vi "Target.vi"() -> ()   [LabVIEW 2018]
uses:
  <vilib>/rvi/Emulation/niFpgaGetClockAttributes.vi
  <vilib>/rvi/Emulation/niFpgaSctlEmulationGetInTimedLoop.vi
  <vilib>/rvi/Emulation/niFpgaEmulationReportErrorSimple.vi
  <vilib>/rvi/eio/common/nirviEmuTemplateMethod_errors.vi
  <vilib>/rvi/Emulation/niFpgaCriticalErrorInLSC.vi
  <vilib>/eio/EIONode/EIONode.xnode
panel:
  out "DAT":bool[](array[boolean])
  in  "CLK":i32=20
  in  "CLKDAT ticks":u16=40 caption="Count(Ticks)"
  in  "CLKDAT":bool
  in  "Частота":bool
  out "MISO":bool[](array[boolean])
  in  "Offset":i16=-1
  in  "phase offset N":fxp<+,32,0>=0.25
  in  "frequency N":fxp<+,32,0>=2.491287887096405e-08
  in  "phase offset P":fxp<+,32,0>
  in  "frequency P":fxp<+,32,0>=2.491287887096405e-08
  in  "N (24/16)":i32=24
  in  "MOSI":bool[](array[boolean])=[FALSE, FALSE, FALSE, FALSE, FALSE, FALSE, FALSE, FALSE, FALSE, FALSE, FALSE, FALSE, FALSE, FALSE, FALSE, FALSE, FALSE, FALSE, FALSE, FALSE, FALSE, FALSE, FALSE, FALSE]
  in  "Count(Ticks)":u16=40
  in  "NPRG":bool
  out "NERR":bool
  out "INCB":bool
  out "INCA":bool
  out "B":bool
  out "A":bool
  out "Z":bool
  out "INCZ":bool
  out "PSIN":i16
  out "POK":i16
  out "ERR":i16
  out "NCOS":i16
  out "NSIN":i16
  out "PCOS":i16
  in  "Регистр":bool
  in  "Стоп":bool
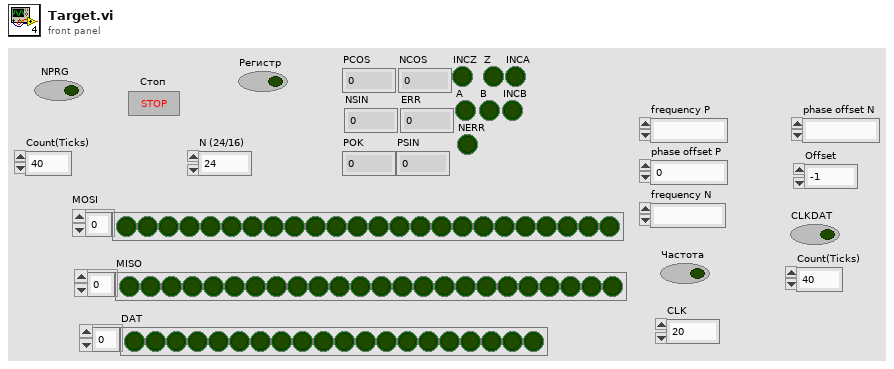
[diagram p1: front panel]
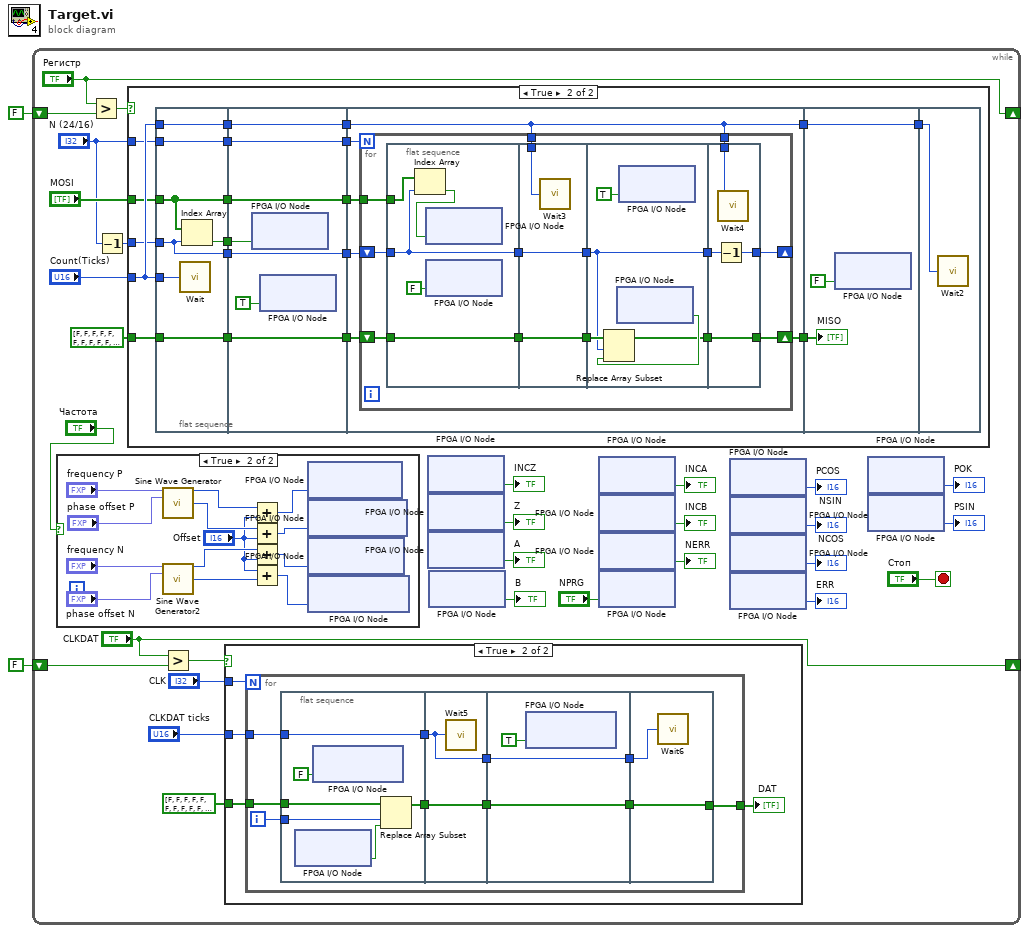
[diagram p0: block diagram]
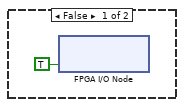
[diagram p2: hidden frame]
diagram:
  n1 = while {
    shift-right: ["CLKDAT"] -> _
    shift-left: FALSE ("CLKDAT") -> [w8]
    shift-right: ["Регистр"] -> _
    shift-left: FALSE ("Регистр") -> [w5]
    stop <- "Стоп" stop-if-true
    n2 = case shown="True" "Частота" {
      frame False {
      }
      frame True {
        n3 = call "Sine Wave Generator"("frequency (periods/tick)"="frequency P", "phase offset (periods)"="phase offset P") -> ("sine out"=w69:i16, "cosine out"=w68:i16)  [unwired: 12 in]
        n4 = call "Sine Wave Generator2"("frequency (periods/tick)"="frequency N", "phase offset (periods)"="phase offset N") -> ("sine out"=w67:i16, "cosine out"=w66:i16)  [unwired: 12 in]
        n5 = Add(x=w69, y="Offset") -> (x+y=w64:i16)
        n6 = Add(x=w68, y="Offset") -> (x+y=w63:i16)
        n7 = Add(x=w67, y="Offset") -> (x+y=w62:i16)
        n8 = Add(x="Offset", y=w66) -> (x+y=w61:i16)
        n9 = xnode "FPGA I/O Node"("PSIN_NQI"=w64) -> ()  [unwired: 1 in, 1 out]
        n10 = xnode "FPGA I/O Node"("PCOS_NQI"=w63) -> ()  [unwired: 1 in, 1 out]
        n11 = xnode "FPGA I/O Node"("NSIN_NQI"=w62) -> ()  [unwired: 1 in, 1 out]
        n12 = xnode "FPGA I/O Node"("NCOS_NQI"=w61) -> ()  [unwired: 1 in, 1 out]
      }
    }
    n13 = Greater?(x="Регистр", y=w5) -> (0:w3:bool)
    n14 = Decrement(x="N (24/16)") -> (x-1=w13:i32)
    n15 = case shown="True" w3 {
      tunnel: "Count(Ticks)" -> [_ w92]
      tunnel: w13 -> [_ w91]
      tunnel: "MOSI" -> [_ w90]
      tunnel: bool[] [FALSE, FALSE, FALSE, FALSE, FALSE, FALSE, FALSE, FALSE, FALSE, FALSE, FALSE, FALSE, FALSE, FALSE, FALSE, FALSE, FALSE, FALSE, FALSE, FALSE, FALSE, FALSE, FALSE, FALSE] ("MISO") -> [_ w89]
      tunnel: "N (24/16)" -> [_ w76]
      frame False {
      }
      frame True {
        n16 = flat-sequence {
          tunnel: w92 -> [w99]
          tunnel: [w98] -> w88
          tunnel: w92 -> [w98]
          tunnel: [w97] -> w87
          tunnel: w91 -> [w96]
          tunnel: [w96] -> w86
          tunnel: w90 -> [w95]
          tunnel: [w95] -> w85
          tunnel: [w94] -> w84
          tunnel: w89 -> [w94]
          tunnel: [w93] -> w77
          tunnel: w76 -> [w93]
          tunnel: [w105] -> w83
          tunnel: w88 -> [w105]
          tunnel: w87 -> [w102]
          tunnel: w86 -> [w104]
          tunnel: [w104] -> w82
          tunnel: [w103] -> w81
          tunnel: w85 -> [w103]
          tunnel: [w101] -> w80
          tunnel: w84 -> [w101]
          tunnel: w77 -> [w100]
          tunnel: [w100] -> w75
          tunnel: [w111] -> w79
          tunnel: w83 -> [w111]
          tunnel: w82 -> [w109]
          tunnel: w81 -> [w112]
          tunnel: w80 -> [w110]
          tunnel: w75 -> [w108]
          tunnel: [w107] -> w74
          tunnel: [w144] -> w78
          tunnel: w79 -> [w144]
          tunnel: w74 -> [w143]
          tunnel: w78 -> [w146]
          frame #0 {
            n17 = call "Wait"("Count(Ticks)"=w99) -> ()  [unwired: 1 out]
            n18 = Index Array(array=w95, index=w96) -> (element=w97:bool)
          }
          frame #1 {
            n19 = xnode "FPGA I/O Node"("MOSI"=w102) -> ()  [unwired: 1 in, 1 out]
            n20 = xnode "FPGA I/O Node"("CS"=TRUE) -> ()  [unwired: 1 in, 1 out]
          }
          frame #2 {
            n21 = for {
              N: w108 -> [_]
              tunnel: w111 -> [w125]
              shift-right: [w120] -> _
              shift-left: w109 -> [w124]
              tunnel: w112 -> [w122]
              tunnel: w111 -> [w121]
              shift-right: [w114] -> w107
              shift-left: w110 -> [w119]
              n22 = flat-sequence {
                tunnel: w124 -> [w128]
                tunnel: [w128] -> w123
                tunnel: w122 -> [w129]
                tunnel: w119 -> [w126]
                tunnel: [w126] -> w115
                tunnel: w125 -> [w133]
                tunnel: w123 -> [w132]
                tunnel: [w132] -> w117
                tunnel: [w131] -> w116
                tunnel: w115 -> [w131]
                tunnel: [w135] -> w118
                tunnel: w117 -> [w135]
                tunnel: w116 -> [w136]
                tunnel: [w134] -> w113
                tunnel: w121 -> [w142]
                tunnel: [w141] -> w120
                tunnel: w118 -> [w140]
                tunnel: [w139] -> w114
                tunnel: w113 -> [w139]
                frame #0 {
                  n23 = Index Array(array=w129, index=w128) -> (element=w127:bool)
                  n24 = xnode "FPGA I/O Node"("MOSI"=w127) -> ()  [unwired: 1 in, 1 out]
                  n25 = xnode "FPGA I/O Node"("SCK"=FALSE) -> ()  [unwired: 1 in, 1 out]
                }
                frame #1 {
                  n26 = call "Wait3"("Count(Ticks)"=w133) -> ()  [unwired: 1 out]
                }
                frame #2 {
                  n27 = xnode "FPGA I/O Node"() -> ("MISO"=w137:bool)  [unwired: 1 in, 1 out]
                  n28 = Replace Array Subset(array=w136, new element=w137, index=w135) -> (w134:bool[])
                  n29 = xnode "FPGA I/O Node"("SCK"=TRUE) -> ()  [unwired: 1 in, 1 out]
                }
                frame #3 {
                  n30 = Decrement(x=w140) -> (x-1=w141:i32)
                  n31 = call "Wait4"("Count(Ticks)"=w142) -> ()  [unwired: 1 out]
                }
              }
            }
          }
          frame #3 {
            n32 = xnode "FPGA I/O Node"("CS"=FALSE) -> ()  [unwired: 1 in, 1 out]
            "MISO" <- w143
          }
          frame #4 {
            n33 = call "Wait2"("Count(Ticks)"=w146) -> ()  [unwired: 1 out]
          }
        }
      }
    }
    n34 = Greater?(x="CLKDAT", y=w8) -> (0:w7:bool)
    n35 = case shown="True" w7 {
      tunnel: "CLKDAT ticks" -> [_ w37]
      tunnel: "CLK" -> [_ w36]
      tunnel: bool[] [FALSE, FALSE, FALSE, FALSE, FALSE, FALSE, FALSE, FALSE, FALSE, FALSE, FALSE, FALSE, FALSE, FALSE, FALSE, FALSE, FALSE, FALSE, FALSE, FALSE] ("DAT") -> [_ w35]
      frame False {
        n36 = xnode "FPGA I/O Node"("CLK_NQI"=TRUE) -> ()  [unwired: 1 in, 1 out]
      }
      frame True {
        n37 = for {
          N: w36 -> [_]
          tunnel: w37 -> [w44]
          tunnel: w35 -> [w43]
          tunnel: [w38] -> w34
          i -> [w42]
          n38 = flat-sequence {
            tunnel: w44 -> [w53]
            tunnel: [w53] -> w47
            tunnel: w43 -> [w50]
            tunnel: w42 -> [w51]
            tunnel: [w49] -> w39
            tunnel: w47 -> [w55]
            tunnel: [w55] -> w46
            tunnel: [w54] -> w40
            tunnel: w39 -> [w54]
            tunnel: [w57] -> w45
            tunnel: w46 -> [w57]
            tunnel: [w56] -> w41
            tunnel: w40 -> [w56]
            tunnel: w45 -> [w60]
            tunnel: [w59] -> w38
            tunnel: w41 -> [w59]
            frame #0 {
              n39 = xnode "FPGA I/O Node"() -> ("DAT"=w52:bool)  [unwired: 1 in, 1 out]
              n40 = xnode "FPGA I/O Node"("CLK_NQI"=FALSE) -> ()  [unwired: 1 in, 1 out]
              n41 = Replace Array Subset(array=w50, new element=w52, index=w51) -> (w49:bool[])
            }
            frame #1 {
              n42 = call "Wait5"("Count(Ticks)"=w55) -> ()  [unwired: 1 out]
            }
            frame #2 {
              n43 = xnode "FPGA I/O Node"("CLK_NQI"=TRUE) -> ()  [unwired: 1 in, 1 out]
            }
            frame #3 {
              n44 = call "Wait6"("Count(Ticks)"=w60) -> ()  [unwired: 1 out]
            }
          }
        }
        "DAT" <- w34
      }
    }
    n45 = xnode "FPGA I/O Node"() -> ("INCZ"=→"INCZ":bool)  [unwired: 1 in, 1 out]
    n46 = xnode "FPGA I/O Node"() -> ("Z"=→"Z":bool)  [unwired: 1 in, 1 out]
    n47 = xnode "FPGA I/O Node"() -> ("A"=→"A":bool)  [unwired: 1 in, 1 out]
    n48 = xnode "FPGA I/O Node"() -> ("B"=→"B":bool)  [unwired: 1 in, 1 out]
    n49 = xnode "FPGA I/O Node"() -> ("INCA"=→"INCA":bool)  [unwired: 1 in, 1 out]
    n50 = xnode "FPGA I/O Node"() -> ("INCB"=→"INCB":bool)  [unwired: 1 in, 1 out]
    n51 = xnode "FPGA I/O Node"() -> ("NERR"=→"NERR":bool)  [unwired: 1 in, 1 out]
    n52 = xnode "FPGA I/O Node"("NPRG"="NPRG") -> ()  [unwired: 1 in, 1 out]
    n53 = xnode "FPGA I/O Node"() -> ("PCOS"=→"PCOS":i16)  [unwired: 1 in, 1 out]
    n54 = xnode "FPGA I/O Node"() -> ("NSIN"=→"NSIN":i16)  [unwired: 1 in, 1 out]
    n55 = xnode "FPGA I/O Node"() -> ("NCOS"=→"NCOS":i16)  [unwired: 1 in, 1 out]
    n56 = xnode "FPGA I/O Node"() -> ("ERR"=→"ERR":i16)  [unwired: 1 in, 1 out]
    n57 = xnode "FPGA I/O Node"() -> ("POK"=→"POK":i16)  [unwired: 1 in, 1 out]
    n58 = xnode "FPGA I/O Node"() -> ("PSIN"=→"PSIN":i16)  [unwired: 1 in, 1 out]
  }
